vi "Startup_UpdatePathVariables.vi"(8 "error in (no error)":errorcluster, 9 "Message Steps Ref In":refnum<vi>, 10 "MainVI Path":path, 11 "MainFolder Path":path) -> (0 "error out":errorcluster, 1 "Message Steps Ref Out":refnum<vi>, 3 "Paths":T1)   [LabVIEW 2016]
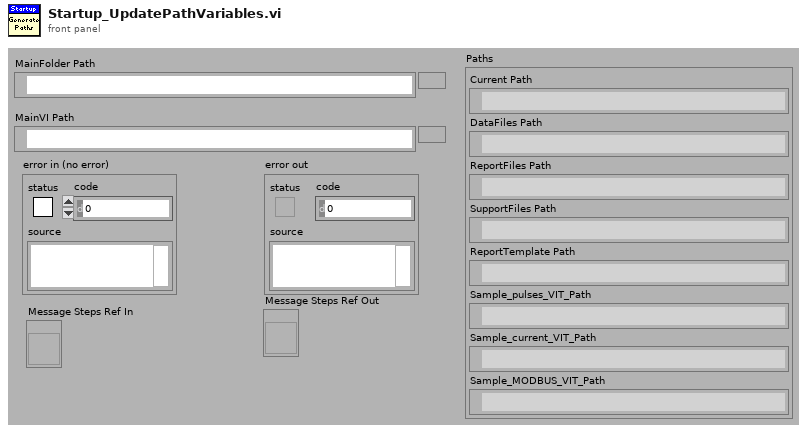
[diagram p1: front panel]
types:
  T1 = cluster{"Current Path":path, "DataFiles Path":path, "ReportFiles Path":path, "SupportFiles Path":path, "ReportTemplate Path":path, "Sample_pulses_VIT_Path":path, "Sample_current_VIT_Path":path, "Sample_MODBUS_VIT_Path":path}
  T2 = cluster{"MainFolder Path":path, "appended path":path, "appended path":path, "appended path":path, "appended path":path, "appended path":path, "appended path":path, "appended path":path}
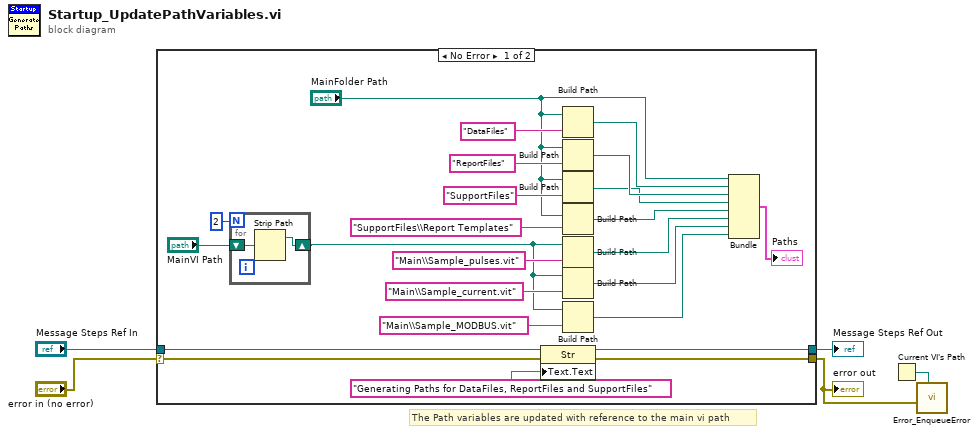
[diagram p0: block diagram]
diagram:
  # "The Path variables are updated with reference to the main vi path"
  n1 = case shown="No Error" "error in (no error)" {
    selector: "error in (no error)" -> [w21 w33]
    tunnel: [w20 w33] -> w1
    tunnel: "Message Steps Ref In" -> [w18 w32]
    tunnel: [w17 w32] -> w3
    frame No Error {
      n2 = for {
        N: 2 -> [_]
        shift-right: [w30] -> w6
        shift-left: "MainVI Path" -> [w31]
        n3 = Strip Path(path=w31) -> (stripped path=w30:path)  [unwired: 1 out]
      }
      n4 = property class="Str"(reference=w18, error in=w21, "Text.Text"="Generating Paths for DataFiles, ReportFiles and SupportFiles") -> (reference out=w17:refnum<vi>, error out=w20:errorcluster)
      n5 = Build Path(base path="MainFolder Path", name or relative path="DataFiles") -> (appended path=w26:path)
      n6 = Build Path(base path="MainFolder Path", name or relative path="ReportFiles") -> (appended path=w25:path)
      n7 = Build Path(base path="MainFolder Path", name or relative path="SupportFiles") -> (appended path=w24:path)
      n8 = Build Path(base path="MainFolder Path", name or relative path="SupportFiles\\Report Templates") -> (appended path=w11:path)
      n9 = Build Path(base path=w6, name or relative path="Main\\Sample_pulses.vit") -> (appended path=w22:path)
      n10 = Build Path(base path=w6, name or relative path="Main\\Sample_current.vit") -> (appended path=w15:path)
      n11 = Build Path(base path=w6, name or relative path="Main\\Sample_MODBUS.vit") -> (appended path=w13:path)
      n12 = Bundle("MainFolder Path"="MainFolder Path", "appended path"=w26, "appended path"=w25, "appended path"=w24, "appended path"=w11, "appended path"=w22, "appended path"=w15, "appended path"=w13) -> (→"Paths":T2)  [unwired: 1 out]
    }
    frame Error {
    }
  }
  "error out" <- w1
  "Message Steps Ref Out" <- w3
  n13 = Current VI's Path() -> (path=w2:path)
  n14 = call "Error_EnqueueError.vi"("SourcePath"=w2, "Error in"=w1) -> ()  [unwired: 1 in, 9 out]
